vi "IsPointInAllyGoalieArea.vi"(8 "error in (no error)":errorcluster, 10 "Point":dbl[](array[numeric]), 11 "Field in":refnum<class "Field.lvclass">) -> (0 "error out":errorcluster, 2 "InGoalieArea":bool, 3 "Field out":refnum<class "Field.lvclass">)   [LabVIEW 2023, in "Field.lvclass"]
uses:
  Field.lvclass
  Field.lvclass/Field.ctl
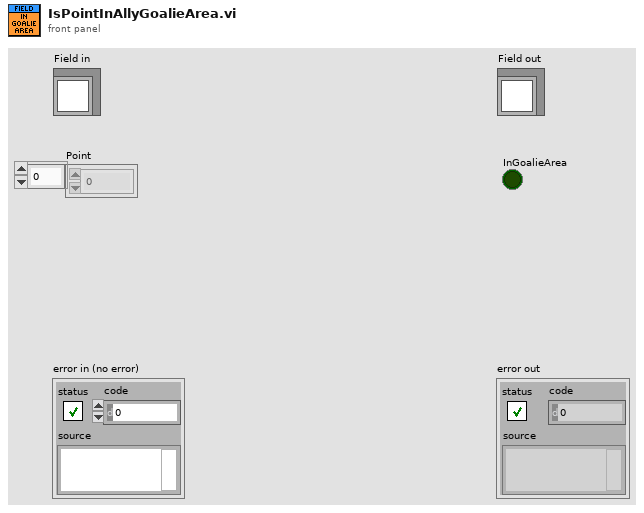
[diagram p1: front panel]
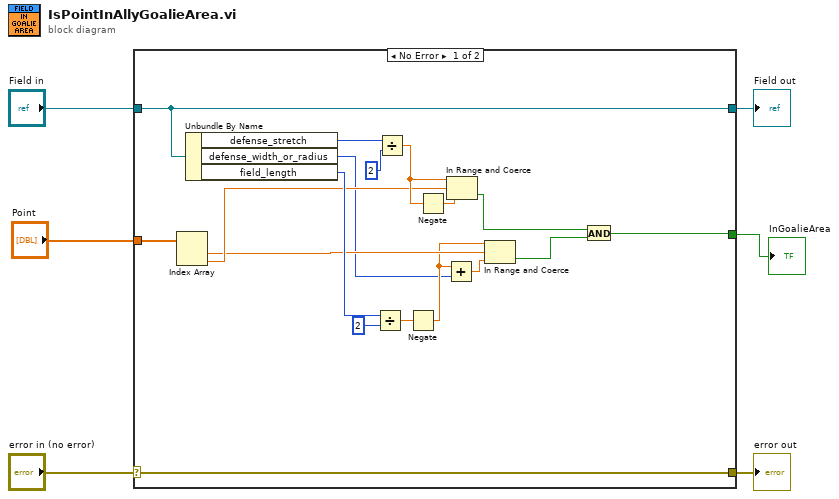
[diagram p0: block diagram]
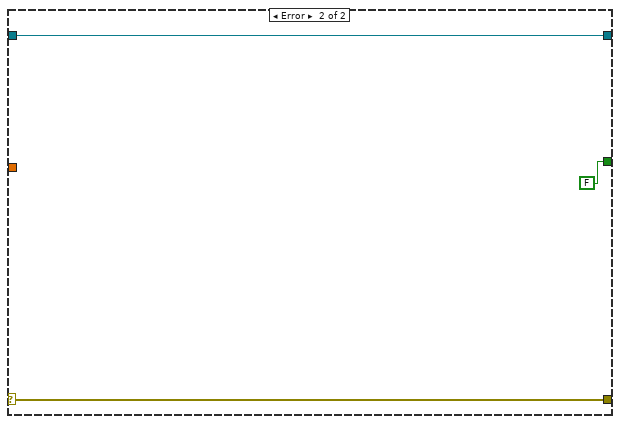
[diagram p2: hidden frame]
diagram:
  n1 = case shown="No Error" "error in (no error)" {
    selector: "error in (no error)" -> [w24 w27]
    tunnel: [w24 w27] -> w5
    tunnel: [w23 w26] -> w3
    tunnel: "Field in" -> [w23 w26]
    tunnel: "Point" -> [w19 _]
    tunnel: [w7 FALSE] -> w1
    frame No Error {
      n2 = Index Array(array=w19) -> (element #1=w14:dbl, element #2=w15:dbl)  [unwired: 2 in]
      n3 = Unbundle By Name(w23) -> ("defense_stretch"=w18:i32, "defense_width_or_radius"=w10:i32, "field_length"=w16:i32)
      n4 = Divide(x=w16, y=2) -> (x/y=w11:dbl)
      n5 = Divide(x=w18, y=2) -> (x/y=w21:dbl)
      n6 = Negate(x=w11) -> (-x=w13:dbl)
      n7 = Negate(x=w21) -> (-x=w20:dbl)
      n8 = Add(x=w13, y=w10) -> (x+y=w12:dbl)
      n9 = In Range and Coerce(upper limit=w21, x=w15, lower limit=w20) -> (In Range?=w9:bool)  [unwired: 1 out]
      n10 = In Range and Coerce(upper limit=w13, x=w14, lower limit=w12) -> (In Range?=w8:bool)  [unwired: 1 out]
      n11 = And(x=w9, y=w8) -> (x .and. y?=w7:bool)
    }
    frame Error {
    }
  }
  "error out" <- w5
  "Field out" <- w3
  "InGoalieArea" <- w1
